vi "Basic Example RT Code.vi"() -> ()   [LabVIEW 2014]
uses:
  <vilib>/rvi/interface/nirviOpenFPGA/nirviOpenFPGA.xnode
  Basic Example.vi
  <vilib>/rvi/interface/nirviReadWriteControl/nirviReadWriteControl.xnode
  NiFpgaLv.dll
  <vilib>/Utility/error.llb/Error Cluster From Error Code.vi
  <vilib>/rvi/interface/Simulation/niFpgaSimulationCallBeginRW.vi
  <vilib>/rvi/errors/niLvFpgaAdjustHostInterfaceError.vi
  <vilib>/rvi/interface/nirviMethod/nirviMethod.xnode
  <vilib>/FPGAPlugInAG/Dynamic/niLvFpga_ReadFifo_Dynamic.vi
  <vilib>/rvi/errors/niLvFpgaMergeErrorWithErrorCode.vi
  <vilib>/rvi/interface/nirviCloseFPGA/nirviCloseFPGA.xnode
  <vilib>/FPGAPlugInAG/Dynamic/niLvFpga_Close_Dynamic.vi
panel:
  in  "stop":bool
  out "Waveform Graph":u64[](graph)
  in  "Chip Select":u8
  in  "SPI Command":u64
  in  "data rate (S/s)":u32
  in  "SPI PHY Settings":T1
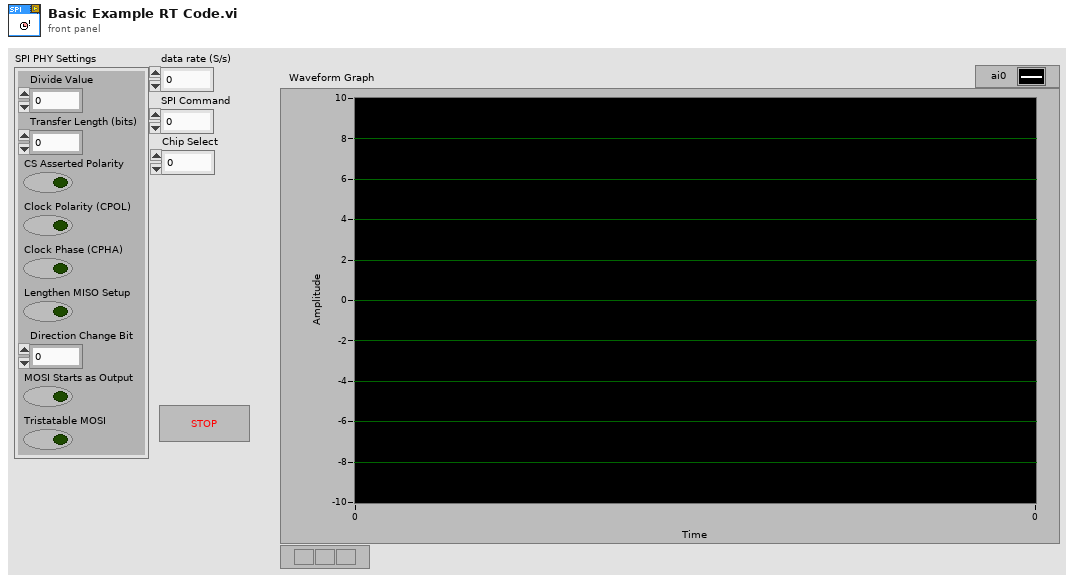
[diagram p1: front panel]
types:
  T1 = cluster{"Divide Value":u8, "Transfer Length (bits)":u8, "CS Asserted Polarity":bool, "Clock Polarity (CPOL)":bool, "Clock Phase (CPHA)":bool, "Lengthen MISO Setup":bool, "Direction Change Bit":u8, "MOSI Starts as Output":bool, "Tristatable MOSI":bool}
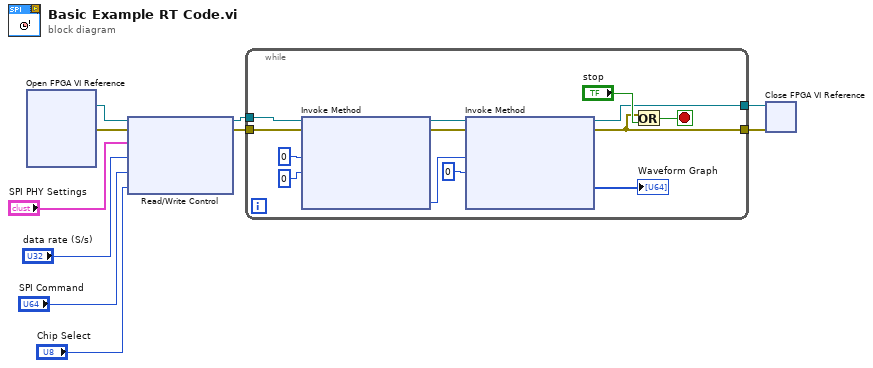
[diagram p0: block diagram]
diagram:
  n1 = xnode "Open FPGA VI Reference"() -> ("FPGA VI Reference Out"=w10:refnum<k20>, "error out"=w9:errorcluster)  [unwired: 2 in]
  n2 = xnode "Read/Write Control"("FPGA VI Reference In"=w10, "error in"=w9, "SPI PHY Settings"="SPI PHY Settings", "data rate (S/s)"="data rate (S/s)", "SPI Command"="SPI Command", "Chip Select"="Chip Select") -> ("FPGA VI Reference Out"=w6:refnum<k20>, "error out"=w5:errorcluster)
  n3 = while {
    tunnel: w6 -> [w23]
    tunnel: w5 -> [w16]
    tunnel: [w12] -> w2
    tunnel: [w11] -> w1
    stop <- w14 stop-if-true
    n4 = xnode "Invoke Method"("FPGA VI Reference In"=w23, "error in"=w16, "Number of Elements"=u32 0, "Timeout (ms)"=0) -> ("FPGA VI Reference Out"=w22:refnum<k20>, "error out"=w15:errorcluster, "Elements Remaining"=w19:u32)  [unwired: 1 out]
    n5 = xnode "Invoke Method"("FPGA VI Reference In"=w22, "error in"=w15, "Number of Elements"=w19, "Timeout (ms)"=0) -> ("FPGA VI Reference Out"=w11:refnum<k20>, "error out"=w12:errorcluster, "Data"=→"Waveform Graph":u64[])  [unwired: 1 out]
    n6 = Or(x=w12, y="stop") -> (x .or. y?=w14:bool)
  }
  n7 = xnode "Close FPGA VI Reference"("FPGA VI Reference In"=w1, "error in"=w2) -> ()  [unwired: 1 out]
